vi "Set Temp Control--Method.vi"(8 "error in (no error)":errorcluster, 10 "Temp Control":bool, 11 "Simulated Thermal Process Controller in":refnum<class "Simulated Thermal Process Controller.lvclass">) -> (0 "error out":errorcluster, 3 "Simulated Thermal Process Controller out":refnum<class "Simulated Thermal Process Controller.lvclass">)   [LabVIEW 2024, in "Simulated Thermal Process Controller.lvclass"]
uses:
  Simulated Thermal Process Controller.lvclass
  Simulated Thermal Process Controller.lvclass/Simulated Thermal Process Controller.ctl
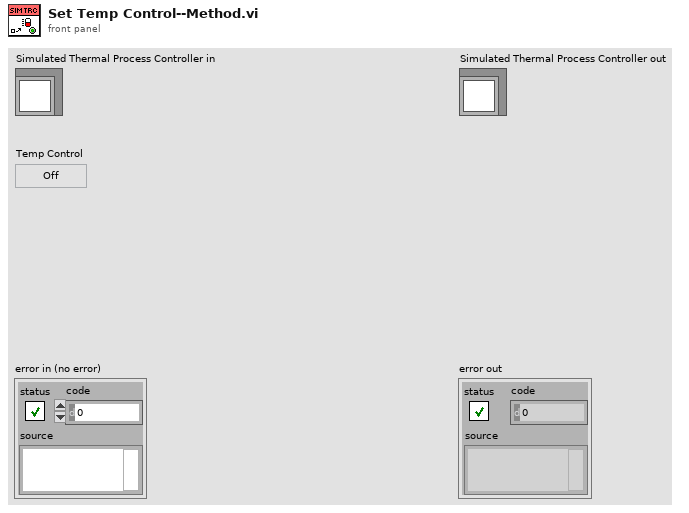
[diagram p1: front panel]
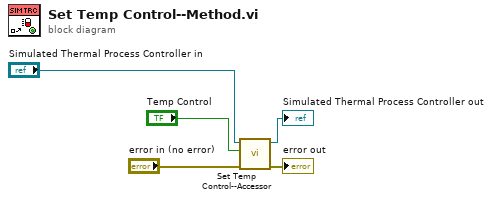
[diagram p0: block diagram]
diagram:
  n1 = call "Set Temp Control--Accessor.vi"("error in (no error)"="error in (no error)", "Temp Control"="Temp Control", "Simulated Thermal Process Controller in"="Simulated Thermal Process Controller in") -> ("error out"=→"error out":errorcluster, "Simulated Thermal Process Controller out"=→"Simulated Thermal Process Controller out":refnum<class "Simulated Thermal Process Controller.lvclass">)  [unwired: 7 in]
